vi "FL_Make_data_frame_and_put_to_queue.vi"(8 "error in":errorcluster, 10 "Queue in":refnum<queue>, 11 "VISA resource name in":refnum<visa-resource-name>) -> (0 "error out":errorcluster, 1 "Timestamp":timestamp, 2 "Queue out":refnum<queue>, 3 "VISA resource name out":refnum<visa-resource-name>, 5 "Read buffer (for reference only, data is queued)":string)   [LabVIEW 2016]
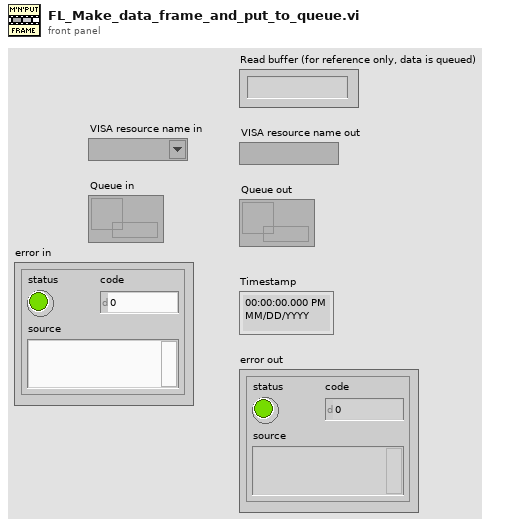
[diagram p1: front panel]
types:
  T1 = cluster{string, "seconds since 1Jan1904":timestamp}
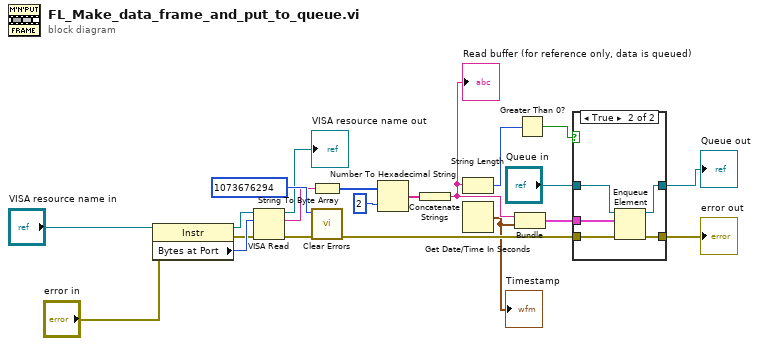
[diagram p0: block diagram]
diagram:
  n1 = property class="Instr"(reference="VISA resource name in", error in="error in") -> (reference out=w3:refnum<visa-resource-name>, error out=w4:errorcluster, "Bytes at Port"=w5:u32)
  n2 = VISA Read(VISA resource name=w3, byte count=w5, error in (no error)=w4) -> (VISA resource name out=→"VISA resource name out":refnum<visa-resource-name>, read buffer=w9:string, error out=w11:errorcluster)  [unwired: 1 out]
  n3 = String To Byte Array(string=w9) -> (unsigned byte array=w7:u8[])
  n4 = call <vilib>:"Clear Errors.vi"("error in (no error)"=w11, "specific error code to clear (0: all)"=1073676294) -> ("error out"=w14:errorcluster)  [unwired: 4 in, 1 out]
  n5 = Number To Hexadecimal String(1:i16 2 ("width (-)"), 2:w7) -> (0:w18:string[])
  n6 = Concatenate Strings(w18) -> (w21:string)
  "Read buffer (for reference only, data is queued)" <- w21
  n7 = String Length(string=w21) -> (length=w19:i32)
  n8 = Get Date/Time In Seconds ("Current time")() -> (seconds since 1Jan1904=w12:timestamp)
  "Timestamp" <- w12
  n9 = Bundle(w21, "seconds since 1Jan1904"=w12) -> (w13:T1)  [unwired: 1 in]
  n10 = Greater Than 0?(x=w19) -> (x > 0?=w20:bool)
  n11 = case shown="True" w20 {
    tunnel: w13 -> [_ w24]
    tunnel: w14 -> [w23 w26]
    tunnel: [w23 w25] -> w15
    tunnel: "Queue in" -> [w22 w28]
    tunnel: [w22 w27] -> w17
    frame False {
    }
    frame True {
      n12 = Enqueue Element(queue=w28, element=w24, error in (no error)=w26) -> (queue out=w27:refnum<queue>, error out=w25:errorcluster)  [unwired: 1 in, 1 out]
    }
  }
  "Queue out" <- w17
  "error out" <- w15
